vi "TagDB Refmgr-Auto Refresh.vi"(7 "DataDB":T1, 8 "error in (no error)":errorcluster, 10 "Rules":T2[](array[typedef]), 11 "DB Ref":T1) -> (0 "error out":errorcluster, 3 "DB Ref (dup)":T1)   [LabVIEW 2017, in "TagDB RefManager.lvlib"]
uses:
  TagDB RefManager.lvlib
  <userlib>/_NEVSTOP/TagDB/Typedef/TagDB.ctl
  Typedef/RefMgr-Logic-State.ctl
  Typedef/RefMgr-StateChangeType.ctl
  ad0d2cce-a5b7-4b1b-8c86-61dd78e8b0b8.vi
  <userlib>/_NEVSTOP/TagDB/TagDB.lvlib
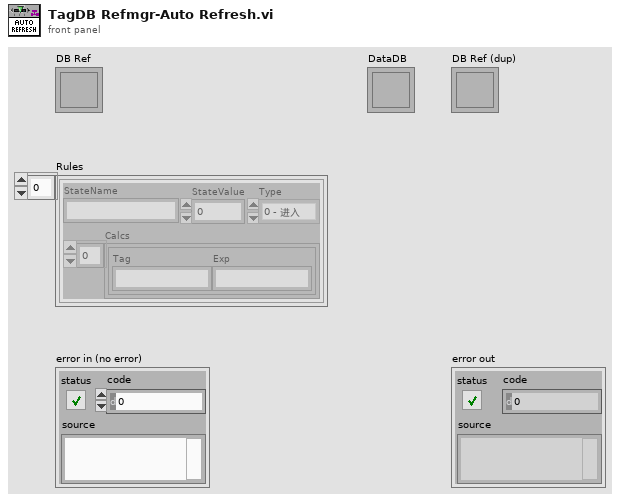
[diagram p1: front panel]
types:
  T1 = typedef "TagDB.lvlib/TagDB.ctl" = refnum<k1>
  T2 = typedef "TagDB RefManager.lvlib/RefMgr-Logic-State.ctl" = cluster{"StateName":string, "StateValue":i32, "Type":T3, "Calcs":cluster{"Tag":string, "Exp":string}[]}
  T3 = typedef "TagDB RefManager.lvlib/RefMgr-StateChangeType.ctl" = enum16{"0 - 进入", "1 - 等于", "2 - 退出"}
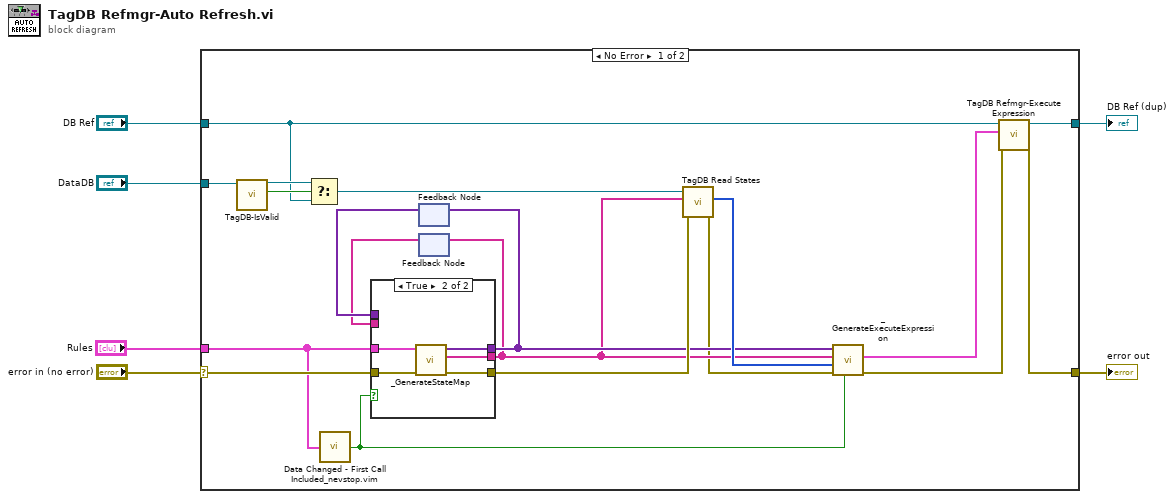
[diagram p0: block diagram]
diagram:
  n1 = case shown="No Error" "error in (no error)" {
    selector: "error in (no error)" -> [w25 w35]
    tunnel: [w19 w35] -> w5
    tunnel: "DB Ref" -> [w9 w34]
    tunnel: [w21 w34] -> w3
    tunnel: "Rules" -> [w17 _]
    tunnel: "DataDB" -> [w24 _]
    frame No Error {
      n2 = call <userlib>:"TagDB-IsValid.vi"("TagDB"=w24) -> ("valid TagDB?"=w11:bool, "TagDB(dup)"=w10:T1)  [unwired: 8 in, 1 out]
      n3 = Select(t=w10, s=w11, f=w9) -> (s? t:f=w8:T1)
      n4 = call "Data Changed - First Call Included_nevstop.vim"("Variant"=w17) -> ("Changed"=w16:bool)
      n5 = feedback #1() -> (w14:variant[])  [unwired: 1 in]
      n6 = feedback #2() -> (w12:string[])  [unwired: 1 in]
      n7 = case shown="True" w16 {
        tunnel: w25 -> [w28 w33]
        tunnel: [w26 w32] -> w15
        tunnel: [w28 w31] -> w23
        tunnel: [w27 w30] -> w13
        tunnel: w17 -> [_ w29]
        tunnel: w14 -> [w26 _]
        tunnel: w12 -> [w27 _]
        frame False {
        }
        frame True {
          n8 = call "_GenerateStateMap.vi"("error in (no error)"=w33, "Rules"=w29) -> ("error out"=w31:errorcluster, "StateNames"=w30:string[], "RulesMap"=w32:variant[])  [unwired: 7 in]
        }
      }
      n9 = feedback-in #1(w15) -> ()
      n10 = feedback-in #2(w13) -> ()
      n11 = call "TagDB Read States.vi"("error in (no error)"=w23, "StateNames"=w13, "Refnum in"=w8) -> ("error out"=w7:errorcluster, "State"=w22:i32[])  [unwired: 6 in, 1 out]
      n12 = call "_GenerateExecuteExpression.vi"("first call?"=w16, "error in (no error)"=w7, "States"=w22, "StateNames"=w13, "RulesMap"=w15) -> ("error out"=w20:errorcluster, "exps"=w18:cluster{"Tag":string, "formula":string}[])  [unwired: 4 in, 1 out]
      n13 = call "TagDB Refmgr-Execute Expression.vi"("error in (no error)"=w20, "expressions"=w18, "DB Ref"=w9) -> ("error out"=w19:errorcluster, "DB Ref (dup)"=w21:T1)  [unwired: 6 in, 1 out]
    }
    frame Error {
    }
  }
  "error out" <- w5
  "DB Ref (dup)" <- w3
